vi "timing harness--json load.vi"() -> ()   [LabVIEW 2021]
uses:
  _Material Theme SubVIs/material theme.ctl
  _Material Theme SubVIs/material json scheme.ctl
  _Material Theme SubVIs/material json palette.ctl
  b89b152c-4396-4218-802e-881716382aa8.vi
  <vilib>/JDP Science/JSONtext/JSON text to Variant.vi
  <vilib>/JDP Science/JSONtext/LVClass Serializer/JSONtext LVClass Serializer.lvclass
  Material Theme/Material Theme.lvclass
panel:
  out "avg per loop (ms)":dbl
  in  "loops":i32=100
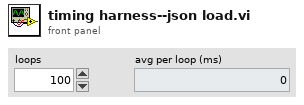
[diagram p1: front panel]
types:
  T1 = typedef "material theme.ctl" = cluster{"description":string, "seed":string, "coreColors":cluster{"primary":string, "secondary":string, "tertiary":string, "error":string}, "schemes":cluster{"light":T2, "light-medium-contrast":T2, "light-high-contrast":T2, "dark":T2, "dark-medium-contrast":T2, "dark-high-contrast":T2}, "palettes":cluster{"primary":T3, "secondary":T3, "tertiary":T3, "neutral":T3, "neutral-variant":T3}}
  T2 = typedef "material json scheme.ctl" = cluster{"primary":string, "surfaceTint":string, "onPrimary":string, "primaryContainer":string, "onPrimaryContainer":string, "secondary":string, "onSecondary":string, "secondaryContainer":string, "onSecondaryContainer":string, "tertiary":string, "onTertiary":string, "tertiaryContainer":string, "onTertiaryContainer":string, "error":string, "onError":string, "errorContainer":string, "onErrorContainer":string, "background":string, "onBackground":string, "surface":string, "onSurface":string, "surfaceVariant":string, "onSurfaceVariant":string, "outline":string, "outlineVariant":string, "shadow":string, "scrim":string, "inverseSurface":string, "inverseOnSurface":string, "inversePrimary":string, "primaryFixed":string, "onPrimaryFixed":string, "primaryFixedDim":string, "onPrimaryFixedVariant":string, "secondaryFixed":string, "onSecondaryFixed":string, "secondaryFixedDim":string, "onSecondaryFixedVariant":string, "tertiaryFixed":string, "onTertiaryFixed":string, "tertiaryFixedDim":string, "onTertiaryFixedVariant":string, "surfaceDim":string, "surfaceBright":string, "surfaceContainerLowest":string, "surfaceContainerLow":string, "surfaceContainer":string, "surfaceContainerHigh":string, "surfaceContainerHighest":string}
  T3 = typedef "material json palette.ctl" = cluster{"0":string, "5":string, "10":string, "15":string, "20":string, "25":string, "30":string, "35":string, "40":string, "50":string, "60":string, "70":string, "80":string, "90":string, "95":string, "98":string, "99":string, "100":string}
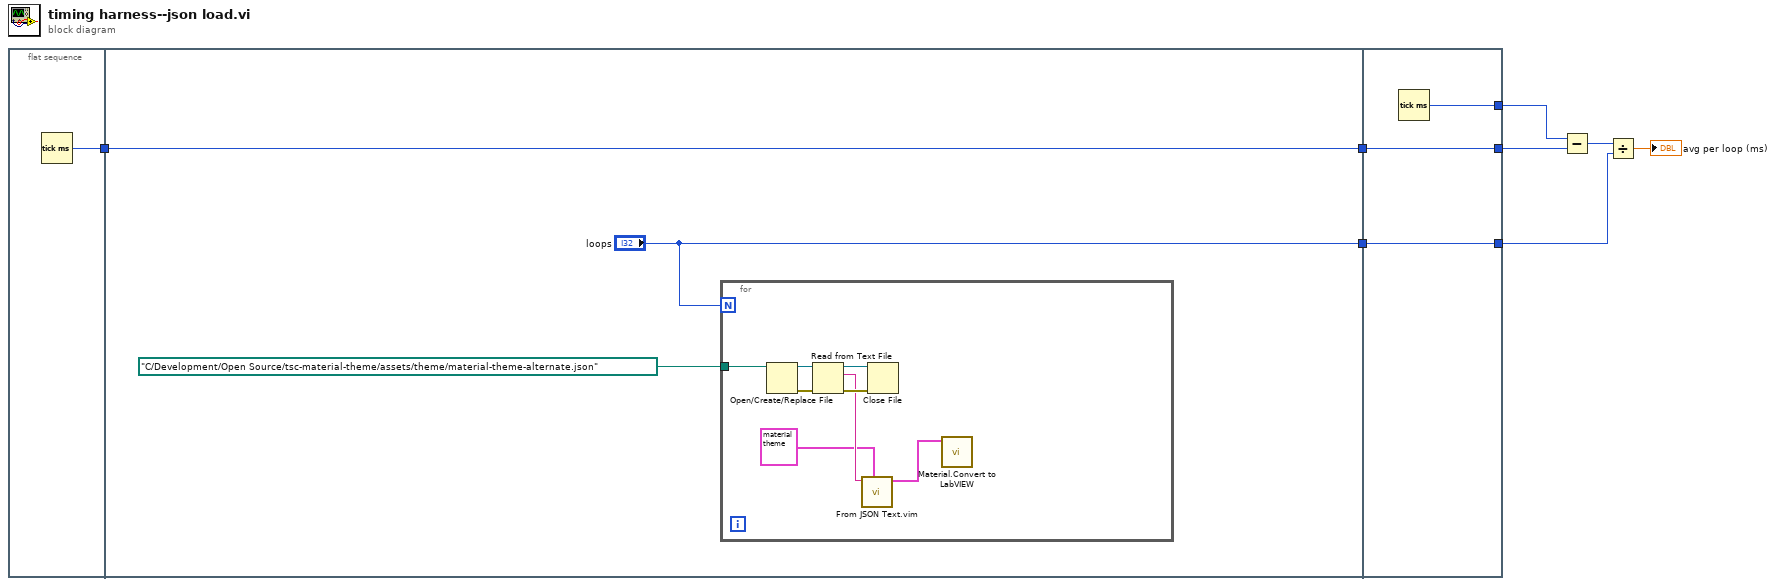
[diagram p0: block diagram]
diagram:
  n1 = flat-sequence {
    tunnel: [w9] -> w8
    tunnel: w8 -> [w11]
    tunnel: [w11] -> w7
    tunnel: ["loops"] -> w3
    tunnel: w7 -> [w23]
    tunnel: [w23] -> w6
    tunnel: [w22] -> w5
    tunnel: w3 -> [w21]
    tunnel: [w21] -> w2
    frame #0 {
      n2 = Tick Count (ms)() -> (millisecond timer value=w9:u32)
    }
    frame #1 {
      n3 = for {
        N: "loops" -> [_]
        tunnel: path "C:/Development/Open Source/tsc-material-theme/assets/theme/material-theme-alternate.json" ("file path (use dialog)") -> [w13]
        n4 = Open/Create/Replace File(file path (use dialog)=w13) -> (refnum out=w17:refnum<file>, error out=w19:errorcluster)  [unwired: 5 in, 1 out]
        n5 = Read from Text File(file (use dialog)=w17, error in=w19) -> (refnum out=w18:refnum<file>, text=w16:string, error out=w20:errorcluster)  [unwired: 2 in, 1 out]
        n6 = call "From JSON Text.vim"("Data Type and Default Value"=T1 {"description"="", "seed"="", "coreColors"={"primary"="", "secondary"="", "tertiary"="", "error"=""}, "schemes"={"light"={"primary"="", "surfaceTint"="", "onPrimary"="", "primaryContainer"="0", "onPrimaryContainer"="0", "secondary"="0", "onSecondary"="0", "secondaryContainer"="0", "onSecondaryContainer"="0", "tertiary"="0", "onTertiary"="0", "tertiaryContainer"="0", "onTertiaryContainer"="0", "error"="0", "onError"="0", "errorContainer"="0", "onErrorContainer"="0", "background"="0", "onBackground"="0", "surface"="0", "onSurface"="0", "surfaceVariant"="0", "onSurfaceVariant"="0", "outline"="0", "outlineVariant"="0", "shadow"="0", "scrim"="0", "inverseSurface"="0", "inverseOnSurface"="0", "inversePrimary"="", "primaryFixed"="0", "onPrimaryFixed"="0", "primaryFixedDim"="0", "onPrimaryFixedVariant"="0", "secondaryFixed"="0", "onSecondaryFixed"="0", "secondaryFixedDim"="0", "onSecondaryFixedVariant"="0", "tertiaryFixed"="0", "onTertiaryFixed"="0", "tertiaryFixedDim"="0", "onTertiaryFixedVariant"="0", "surfaceDim"="0", "surfaceBright"="0", "surfaceContainerLowest"="0", "surfaceContainerLow"="0", "surfaceContainer"="0", "surfaceContainerHigh"="0", "surfaceContainerHighest"="0"}, "light-medium-contrast"={"primary"="", "surfaceTint"="", "onPrimary"="", "primaryContainer"="0", "onPrimaryContainer"="0", "secondary"="0", "onSecondary"="0", "secondaryContainer"="0", "onSecondaryContainer"="0", "tertiary"="0", "onTertiary"="0", "tertiaryContainer"="0", "onTertiaryContainer"="0", "error"="0", "onError"="0", "errorContainer"="0", "onErrorContainer"="0", "background"="0", "onBackground"="0", "surface"="0", "onSurface"="0", "surfaceVariant"="0", "onSurfaceVariant"="0", "outline"="0", "outlineVariant"="0", "shadow"="0", "scrim"="0", "inverseSurface"="0", "inverseOnSurface"="0", "inversePrimary"="", "primaryFixed"="0", "onPrimaryFixed"="0", "primaryFixedDim"="0", "onPrimaryFixedVariant"="0", "secondaryFixed"="0", "onSecondaryFixed"="0", "secondaryFixedDim"="0", "onSecondaryFixedVariant"="0", "tertiaryFixed"="0", "onTertiaryFixed"="0", "tertiaryFixedDim"="0", "onTertiaryFixedVariant"="0", "surfaceDim"="0", "surfaceBright"="0", "surfaceContainerLowest"="0", "surfaceContainerLow"="0", "surfaceContainer"="0", "surfaceContainerHigh"="0", "surfaceContainerHighest"="0"}, "light-high-contrast"={"primary"="", "surfaceTint"="", "onPrimary"="", "primaryContainer"="0", "onPrimaryContainer"="0", "secondary"="0", "onSecondary"="0", "secondaryContainer"="0", "onSecondaryContainer"="0", "tertiary"="0", "onTertiary"="0", "tertiaryContainer"="0", "onTertiaryContainer"="0", "error"="0", "onError"="0", "errorContainer"="0", "onErrorContainer"="0", "background"="0", "onBackground"="0", "surface"="0", "onSurface"="0", "surfaceVariant"="0", "onSurfaceVariant"="0", "outline"="0", "outlineVariant"="0", "shadow"="0", "scrim"="0", "inverseSurface"="0", "inverseOnSurface"="0", "inversePrimary"="", "primaryFixed"="0", "onPrimaryFixed"="0", "primaryFixedDim"="0", "onPrimaryFixedVariant"="0", "secondaryFixed"="0", "onSecondaryFixed"="0", "secondaryFixedDim"="0", "onSecondaryFixedVariant"="0", "tertiaryFixed"="0", "onTertiaryFixed"="0", "tertiaryFixedDim"="0", "onTertiaryFixedVariant"="0", "surfaceDim"="0", "surfaceBright"="0", "surfaceContainerLowest"="0", "surfaceContainerLow"="0", "surfaceContainer"="0", "surfaceContainerHigh"="0", "surfaceContainerHighest"="0"}, "dark"={"primary"="", "surfaceTint"="", "onPrimary"="", "primaryContainer"="0", "onPrimaryContainer"="0", "secondary"="0", "onSecondary"="0", "secondaryContainer"="0", "onSecondaryContainer"="0", "tertiary"="0", "onTertiary"="0", "tertiaryContainer"="0", "onTertiaryContainer"="0", "error"="0", "onError"="0", "errorContainer"="0", "onErrorContainer"="0", "background"="0", "onBackground"="0", "surface"="0", "onSurface"="0", "surfaceVariant"="0", "onSurfaceVariant"="0", "outline"="0", "outlineVariant"="0", "shadow"="0", "scrim"="0", "inverseSurface"="0", "inverseOnSurface"="0", "inversePrimary"="", "primaryFixed"="0", "onPrimaryFixed"="0", "primaryFixedDim"="0", "onPrimaryFixedVariant"="0", "secondaryFixed"="0", "onSecondaryFixed"="0", "secondaryFixedDim"="0", "onSecondaryFixedVariant"="0", "tertiaryFixed"="0", "onTertiaryFixed"="0", "tertiaryFixedDim"="0", "onTertiaryFixedVariant"="0", "surfaceDim"="0", "surfaceBright"="0", "surfaceContainerLowest"="0", "surfaceContainerLow"="0", "surfaceContainer"="0", "surfaceContainerHigh"="0", "surfaceContainerHighest"="0"}, "dark-medium-contrast"={"primary"="", "surfaceTint"="", "onPrimary"="", "primaryContainer"="0", "onPrimaryContainer"="0", "secondary"="0", "onSecondary"="0", "secondaryContainer"="0", "onSecondaryContainer"="0", "tertiary"="0", "onTertiary"="0", "tertiaryContainer"="0", "onTertiaryContainer"="0", "error"="0", "onError"="0", "errorContainer"="0", "onErrorContainer"="0", "background"="0", "onBackground"="0", "surface"="0", "onSurface"="0", "surfaceVariant"="0", "onSurfaceVariant"="0", "outline"="0", "outlineVariant"="0", "shadow"="0", "scrim"="0", "inverseSurface"="0", "inverseOnSurface"="0", "inversePrimary"="", "primaryFixed"="0", "onPrimaryFixed"="0", "primaryFixedDim"="0", "onPrimaryFixedVariant"="0", "secondaryFixed"="0", "onSecondaryFixed"="0", "secondaryFixedDim"="0", "onSecondaryFixedVariant"="0", "tertiaryFixed"="0", "onTertiaryFixed"="0", "tertiaryFixedDim"="0", "onTertiaryFixedVariant"="0", "surfaceDim"="0", "surfaceBright"="0", "surfaceContainerLowest"="0", "surfaceContainerLow"="0", "surfaceContainer"="0", "surfaceContainerHigh"="0", "surfaceContainerHighest"="0"}, "dark-high-contrast"={"primary"="", "surfaceTint"="", "onPrimary"="", "primaryContainer"="0", "onPrimaryContainer"="0", "secondary"="0", "onSecondary"="0", "secondaryContainer"="0", "onSecondaryContainer"="0", "tertiary"="0", "onTertiary"="0", "tertiaryContainer"="0", "onTertiaryContainer"="0", "error"="0", "onError"="0", "errorContainer"="0", "onErrorContainer"="0", "background"="0", "onBackground"="0", "surface"="0", "onSurface"="0", "surfaceVariant"="0", "onSurfaceVariant"="0", "outline"="0", "outlineVariant"="0", "shadow"="0", "scrim"="0", "inverseSurface"="0", "inverseOnSurface"="0", "inversePrimary"="", "primaryFixed"="0", "onPrimaryFixed"="0", "primaryFixedDim"="0", "onPrimaryFixedVariant"="0", "secondaryFixed"="0", "onSecondaryFixed"="0", "secondaryFixedDim"="0", "onSecondaryFixedVariant"="0", "tertiaryFixed"="0", "onTertiaryFixed"="0", "tertiaryFixedDim"="0", "onTertiaryFixedVariant"="0", "surfaceDim"="0", "surfaceBright"="0", "surfaceContainerLowest"="0", "surfaceContainerLow"="0", "surfaceContainer"="0", "surfaceContainerHigh"="0", "surfaceContainerHighest"="0"}}, "palettes"={"primary"={"0"="0", "5"="0", "10"="0", "15"="0", "20"="0", "25"="0", "30"="0", "35"="0", "40"="0", "50"="0", "60"="0", "70"="0", "80"="0", "90"="0", "95"="0", "98"="0", "99"="0", "100"="0"}, "secondary"={"0"="0", "5"="0", "10"="0", "15"="0", "20"="0", "25"="0", "30"="0", "35"="0", "40"="0", "50"="0", "60"="0", "70"="0", "80"="0", "90"="0", "95"="0", "98"="0", "99"="0", "100"="0"}, "tertiary"={"0"="0", "5"="0", "10"="0", "15"="0", "20"="0", "25"="0", "30"="0", "35"="0", "40"="0", "50"="0", "60"="0", "70"="0", "80"="0", "90"="0", "95"="0", "98"="0", "99"="0", "100"="0"}, "neutral"={"0"="0", "5"="0", "10"="0", "15"="0", "20"="0", "25"="0", "30"="0", "35"="0", "40"="0", "50"="0", "60"="0", "70"="0", "80"="0", "90"="0", "95"="0", "98"="0", "99"="0", "100"="0"}, "neutral-variant"={"0"="0", "5"="0", "10"="0", "15"="0", "20"="0", "25"="0", "30"="0", "35"="0", "40"="0", "50"="0", "60"="0", "70"="0", "80"="0", "90"="0", "95"="0", "98"="0", "99"="0", "100"="0"}}}, "JSON"=w16) -> ("Data out"=w14:T1)  [unwired: 8 in, 1 out]
        n7 = Close File(refnum=w18, error in=w20) -> ()  [unwired: 2 out]
        n8 = call "Material.Convert to LabVIEW.vi"("material.json string"=w14) -> ()  [unwired: 10 in, 1 out]
      }
    }
    frame #2 {
      n9 = Tick Count (ms)() -> (millisecond timer value=w22:u32)
    }
  }
  n10 = Subtract(x=w5, y=w6) -> (x-y=w4:u32)
  n11 = Divide(x=w4, y=w2) -> (x/y=→"avg per loop (ms)":dbl)
